vi "avoidRobotModelTestCrash.vi"(7 "time limit(in seconds)\ndefault: 10s":dbl=10.0 format="%#_13g", 8 "error in (no error)":errorcluster, 10 "state in":i32, 11 "Game in":refnum<class "Game.lvclass">) -> (0 "error out":errorcluster, 1 "crash?":bool, 2 "state out":i32, 3 "Game out":refnum<class "Game.lvclass">)   [LabVIEW 2023, in "Game.lvclass"]
uses:
  Game.lvclass
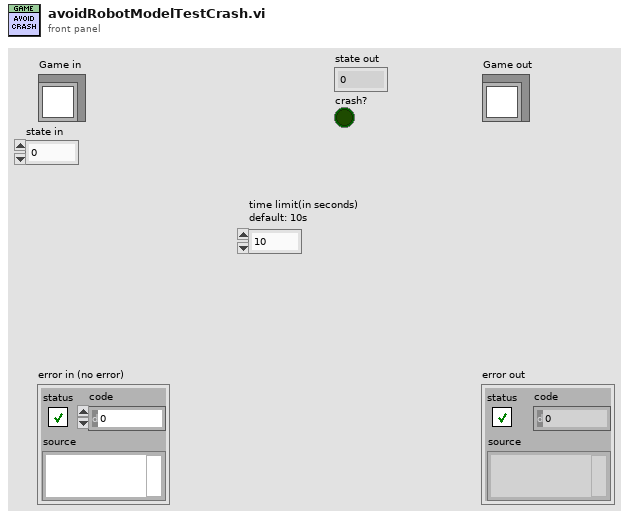
[diagram p1: front panel]
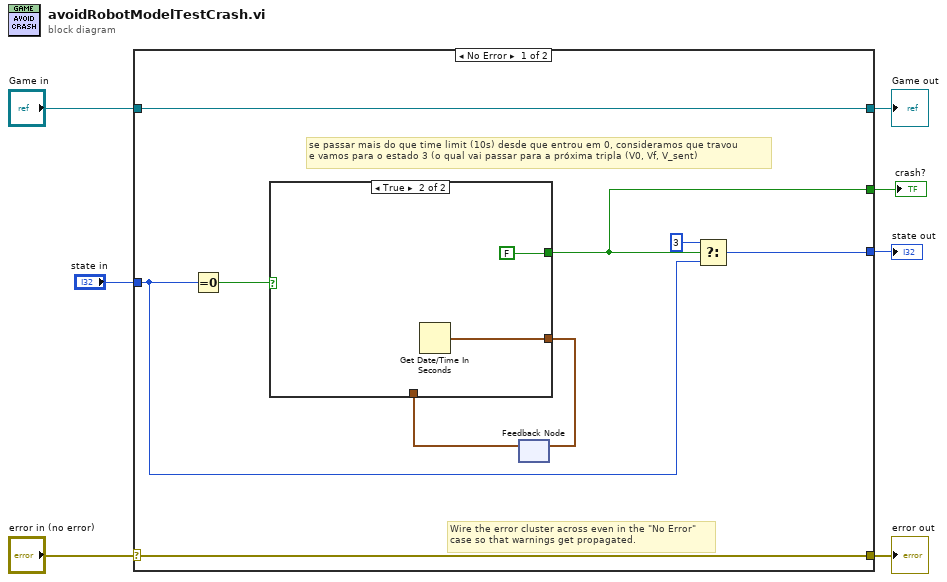
[diagram p0: block diagram]
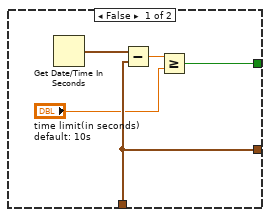
[diagram p2: hidden frame]
diagram:
  n1 = case shown="No Error" "error in (no error)" {
    selector: "error in (no error)" -> [w15 w25]
    tunnel: [w15 w25] -> w6
    tunnel: [w16 w24] -> w4
    tunnel: "Game in" -> [w16 w24]
    tunnel: "state in" -> [w11 _]
    tunnel: [w9 _] -> w2
    tunnel: [w8 _] -> w1
    frame No Error {
      # "se passar mais do que time limit (10s) desde que entrou em 0, consideramos que travou\ne vamos para o estado 3 (o qual vai passar para a próxima tripla (V0, Vf, V_sent)"
      # "Wire the error cluster across even in the \"No Error\"\ncase so that warnings get propagated."
      n2 = Equal To 0?(x=w11) -> (x = 0?=w14:bool)
      n3 = feedback #1() -> (w12:timestamp)  [unwired: 1 in]
      n4 = case shown="True" w14 {
        tunnel: [w20 w23] -> w13
        tunnel: w12 -> [w20 _]
        tunnel: [w18 FALSE] -> w8
        frame False {
          n5 = Get Date/Time In Seconds() -> (seconds since 1Jan1904=w21:timestamp)
          n6 = Subtract(x=w21, y=w20) -> (x-y=w19:dbl)
          n7 = Greater Or Equal?(x=w19, y="time limit(in seconds)\ndefault: 10s") -> (x >= y?=w18:bool)
        }
        frame True {
          n8 = Get Date/Time In Seconds() -> (seconds since 1Jan1904=w23:timestamp)
        }
      }
      n9 = feedback-in #1(w13) -> ()
      n10 = Select(t=3, s=w8, f=w11) -> (s? t:f=w9:i32)
    }
    frame Error {
    }
  }
  "error out" <- w6
  "Game out" <- w4
  "state out" <- w2
  "crash?" <- w1
